vi "CreateCaption.vi"(7 "LaserVariables":string[](array[string]), 8 "WrongScannerRead":string[](array[string]), 9 "WrongLaserVar":string[](array[string]), 10 "WrongVarName":string[](array[string]), 11 "Equal":bool) -> (2 "Caption":string)   [LabVIEW 2016]
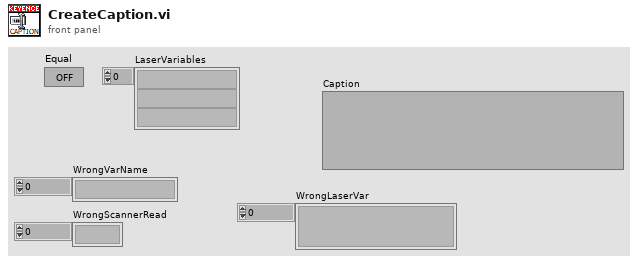
[diagram p1: front panel]
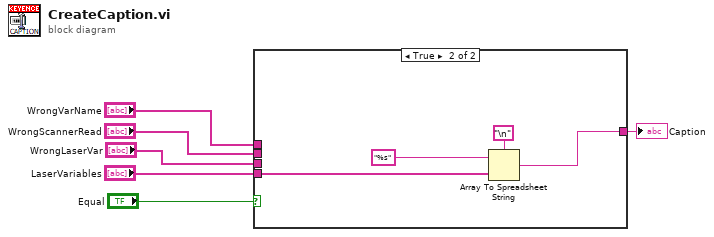
[diagram p0: block diagram]
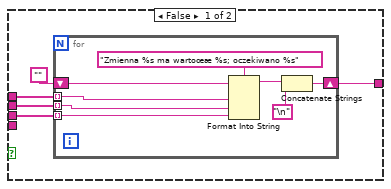
[diagram p2: hidden frame]
diagram:
  n1 = case shown="True" "Equal" {
    tunnel: "LaserVariables" -> [_ w23]
    tunnel: "WrongVarName" -> [w11 _]
    tunnel: "WrongLaserVar" -> [w10 _]
    tunnel: "WrongScannerRead" -> [w9 _]
    tunnel: [w8 w20] -> w6
    frame False {
      n2 = for {
        tunnel: w11 -> [w18] mode=indexing
        tunnel: w10 -> [w17] mode=indexing
        tunnel: w9 -> [w16] mode=indexing
        shift-right: [w13] -> w8
        shift-left: "" -> [w12]
        n3 = Format Into String(format string="Zmienna %s ma wartoœæ %s; oczekiwano %s", initial string=w12, w18, w16, w17) -> (resulting string=w15:string)  [unwired: 1 in, 1 out]
        n4 = Concatenate Strings(w15, "\n") -> (w13:string)
      }
    }
    frame True {
      n5 = Array To Spreadsheet String(delimiter (Tab)="\n", array=w23, 3:"%s" ("format string")) -> (spreadsheet string=w20:string)
    }
  }
  "Caption" <- w6
